vi "Colour Recognition.vi"() -> ()   [LabVIEW 2015]
uses:
  <vilib>/vision/NI_Vision_Development_Module.lvlib
  subVIs/Log Level Control.ctl
  subVIs/Led Control.ctl
  subVIs/Video Resolution Control.ctl
  subVIs/Video Format Control.ctl
  subVIs/Depth Format Control.ctl
  subVIs/Depth Resolution Control.ctl
panel:
  in  "Threshold 2":cluster{"Lower value":sgl, "Upper value":sgl}={"Lower value"=125.0, "Upper value"=160.0} {"Lower value" scale=0.0..255.0; "Upper value" scale=0.0..255.0}
  in  "Led Option":T1
  in  "tilt degree":i32
  in  "Video and Depth config":T6={"Video Resolution"=enum."FREENECT_RESOLUTION_MEDIUM", "Video Format"=enum."FREENECT_VIDEO_RGB", "Depth Format"=enum."FREENECT_DEPTH_11BIT", "Depth Resolution"=enum."FREENECT_RESOLUTION_MEDIUM"}
  in  "Reset Default Settings":bool
  in  "Threshold":cluster{"Lower value":sgl, "Upper value":sgl}={"Lower value"=125.0, "Upper value"=160.0} {"Lower value" scale=0.0..255.0; "Upper value" scale=0.0..255.0}
  in  "Color Recognition":enum16{"Blue", "Red"}(ring)
  out "Image Preview":T7(plugin-control)
  in  "Erosion Value":dbl=5.0
  out "Object Area":dbl
  in  "Area Limit":dbl=2000.0 format="%#_13g"
  out "Colour Matching":T7(plugin-control)
  in  "STOP":bool
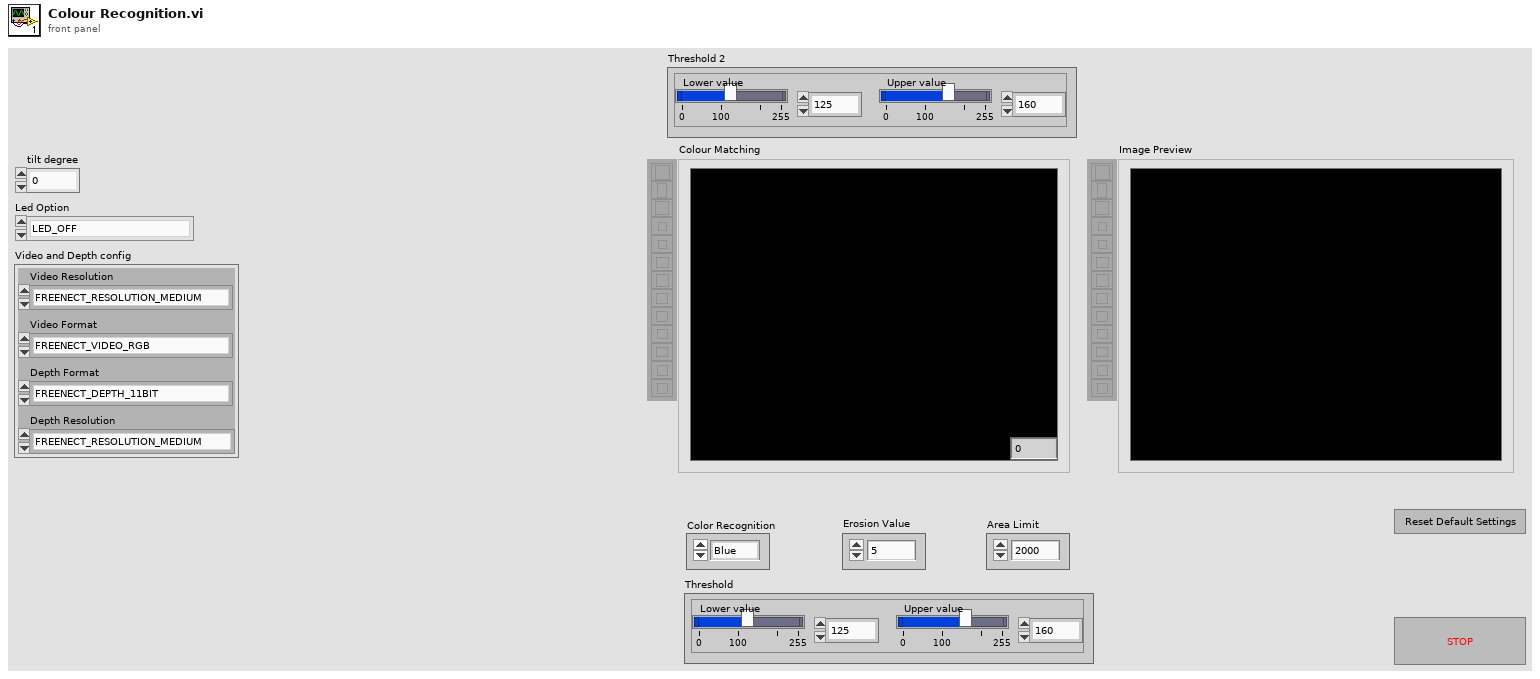
[diagram p1: front panel]
types:
  T1 = typedef "Led Control.ctl" = enum32{"LED_OFF", "LED_GREEN", "LED_RED", "LED_YELLOW", "LED_BLINK_GREEN", "LED_BLINK_GREEN2", "LED_BLINK_RED_YELLOW"}
  T2 = typedef "Video Resolution Control.ctl" = enum32{"FREENECT_RESOLUTION_LOW", "FREENECT_RESOLUTION_MEDIUM", "FREENECT_RESOLUTION_HIGH"}
  T3 = typedef "Video Format Control.ctl" = enum32{"FREENECT_VIDEO_RGB", "FREENECT_VIDEO_BAYER", "FREENECT_VIDEO_IR_8BIT", "FREENECT_VIDEO_IR_10BIT", "FREENECT_VIDEO_IR_10BIT_PACKED", "FREENECT_VIDEO_YUV_RGB", "FREENECT_VIDEO_YUV_RAW"}
  T4 = typedef "Depth Format Control.ctl" = enum32{"FREENECT_DEPTH_11BIT", "FREENECT_DEPTH_10BIT", "FREENECT_DEPTH_11BIT_PACKED", "FREENECT_DEPTH_10BIT_PACKED", "FREENECT_DEPTH_REGISTERED", "FREENECT_DEPTH_MM"}
  T5 = typedef "Depth Resolution Control.ctl" = enum16{"FREENECT_RESOLUTION_TINY", "FREENECT_RESOLUTION_LOW", "FREENECT_RESOLUTION_MEDIUM"}
  T6 = cluster{"Video Resolution":T2, "Video Format":T3, "Depth Format":T4, "Depth Resolution":T5}
  T7 = typedef "IMAQ Image.ctl" = refnum<image>
  T8 = typedef "Log Level Control.ctl" = enum32{"FREENECT_LOG_FATAL", "FREENECT_LOG_ERROR", "FREENECT_LOG_WARNING", "FREENECT_LOG_NOTICE", "FREENECT_LOG_INFO", "FREENECT_LOG_DEBUG", "FREENECT_LOG_SPEW", "FREENECT_LOG_FLOOD"}
  T9 = typedef "Particle Parameters" = i32
  T10 = cluster{"Numeric":dbl, "Numeric":dbl, "Numeric":dbl, "Numeric":dbl}
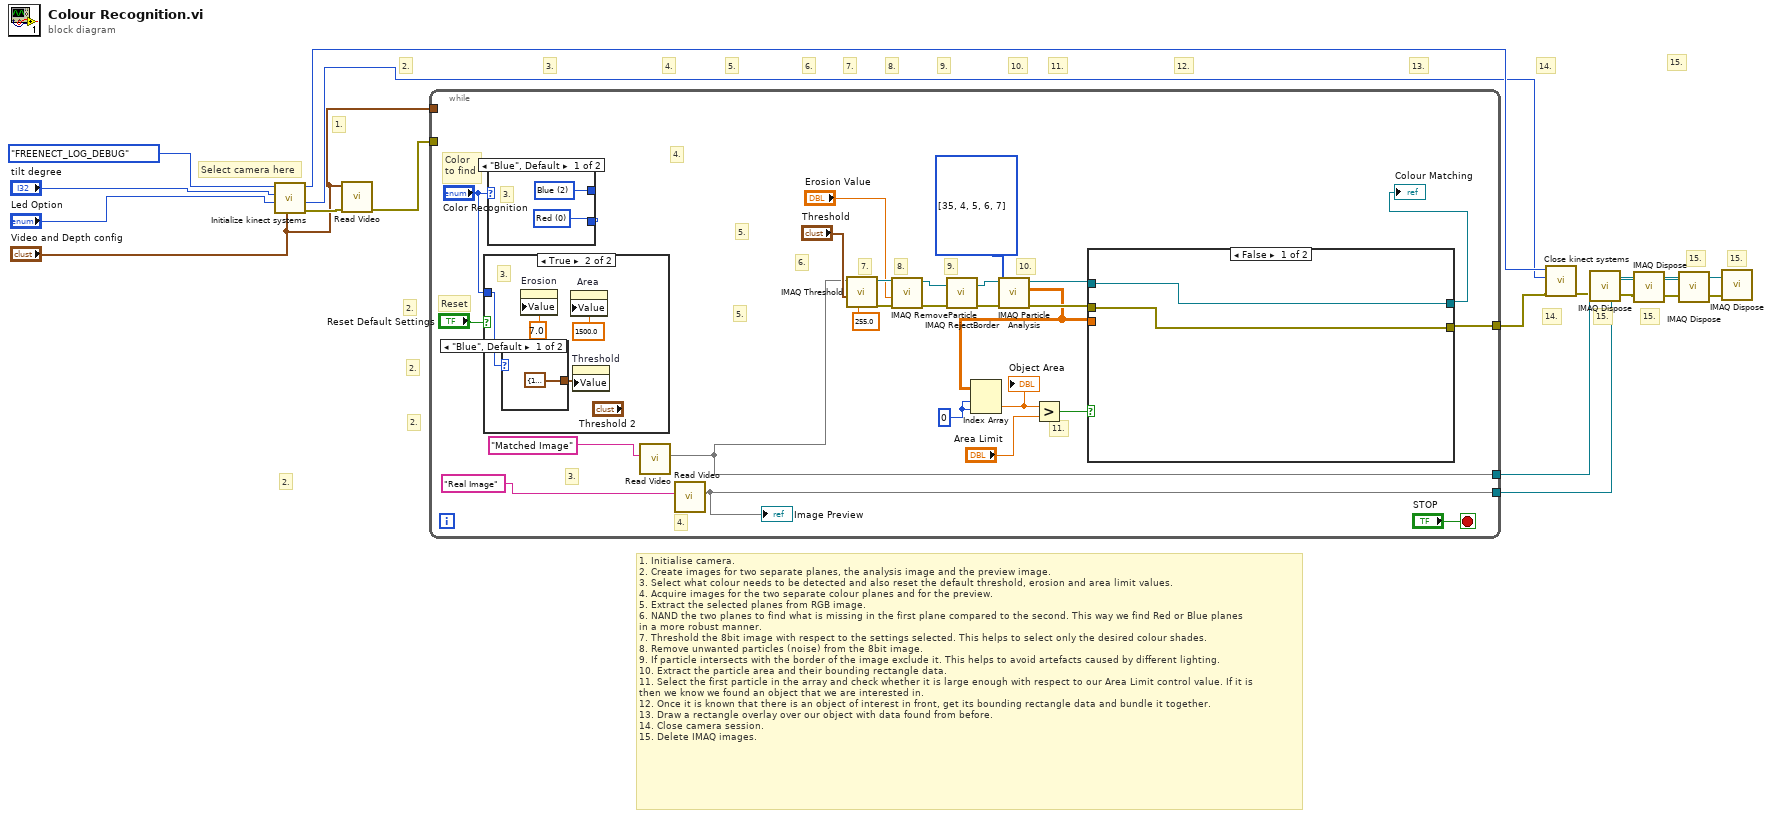
[diagram p0: block diagram]
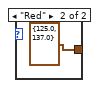
[diagram p3: hidden frame]
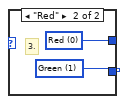
[diagram p4: hidden frame]
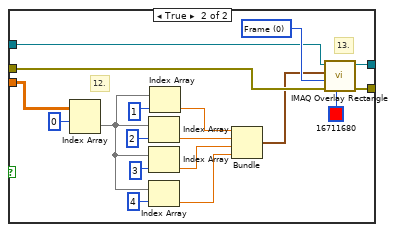
[diagram p5: hidden frame]
diagram:
  # "Select camera here"
  # "1. Initialise camera.\n2. Create images for two separate planes, the analysis image and the preview image.\n3. Select what colour needs to be detected and also reset the default threshold, erosion and area limit values.\n4. Acquire images for the two separate colour planes and for the preview.\n5. Extract the selected planes from RGB image.\n6. NAND the two planes to find what is missing in the first plane compared to the second. This way we find Red or Blue planes\nin a more robust manner.\n7. Threshold the 8bit image with respect to the settings selected. This helps to select only the desired colour shades.\n8. Remove unwanted particles (noise) from the 8bit image.\n9. If particle intersects with the border of the image exclude it. This helps to avoid artefacts caused by different lighting.\n10. Extract the particle area and their bounding rectangle data.\n11. Select the first particle in the array and check whether it is large enough with respect to our Area Limit control value. If it is\nthen we know we found an object that we are interested in.\n12. Once it is known that there is an object of interest in front, get its bounding rectangle data and bundle it together.\n13. Draw a rectangle overlay over our object with data found from before.\n14. Close camera session.\n15. Delete IMAQ images."
  # "15."
  # "15."
  # "15."
  # "15."
  # "15."
  # "14."
  # "14."
  # "13."
  # "12."
  # "11."
  # "10."
  # "2."
  # "2."
  # "2."
  # "2."
  # "9."
  # "8."
  # "7."
  # "6."
  # "5."
  # "4."
  # "3."
  # "2."
  # "1."
  n1 = call "Initialize kinect systems.vi"("Video and Depth config"="Video and Depth config", "Led Option"="Led Option", "tilt degree"="tilt degree", "Log Level"=Log_Level_Control."FREENECT_LOG_DEBUG") -> ("error out"=w3:errorcluster, "Kinect Handle"=w4:i64, "Video Handle out"=w5:i64)  [unwired: 4 in, 1 out]
  n2 = call "Read Video.vi"("error in (no error)"=w3, "input cluster"="Video and Depth config") -> ("error out"=w2:errorcluster)  [unwired: 7 in, 2 out]
  n3 = while {
    tunnel: w2 -> [_]
    tunnel: [w16] -> w13
    tunnel: [w26] -> w6
    tunnel: [w18] -> w11
    tunnel: "Video and Depth config" -> [_]
    stop <- "STOP" stop-if-true
    w37 = 0 ("index (row)")
    w39 = T9[] [35, 4, 5, 6, 7] items=["Center of Mass X", "Center of Mass Y", "First Pixel X", "First Pixel Y", "Bounding Rect Left", "Bounding Rect Top", "Bounding Rect Right", "Bounding Rect Bottom", "Max Feret Diameter Start X", "Max Feret Diameter Start Y", "Max Feret Diameter End X", "Max Feret Diameter End Y", "Max Horiz. Segment Length Left", "Max Horiz. Segment Length Right", "Max Horiz. Segment Length Row", "-", "Bounding Rect Width", "Bounding Rect Height", "Bounding Rect Diagonal", "Perimeter", "Convex Hull Perimeter", "Holes' Perimeter", "Max Feret Diameter", "Equivalent Ellipse Major Axis", "Equivalent Ellipse Minor Axis", "Equivalent Ellipse Minor Axis (Feret)", "Equivalent Rect Long Side", "Equivalent Rect Short Side", "Equivalent Rect Diagonal", "Equivalent Rect Short Side (Feret)", "Average Horiz. Segment Length", "Average Vert. Segment Length", "Hydraulic Radius", "Waddel Disk Diameter", "-", "Area", "Holes' Area", "Particle & Holes' Area", "Convex Hull Area", "Image Area", "-", "Number of Holes", "Number of Horiz. Segments", "Number of Vert. Segments", "-", "Orientation", "Max Feret Diameter Orientation", "-", "% Area/Image Area", "% Area/(Particle & Holes' Area)", "Ratio of Equivalent Ellipse Axes", "Ratio of Equivalent Rect Sides", "-", "Elongation Factor", "Compactness Factor", "Heywood Circularity Factor", "Type Factor", "-", "Sum X", "Sum Y", "Sum XX", "Sum XY", "Sum YY", "Sum XXX", "Sum XXY", "Sum XYY", "Sum YYY", "-", "Moment of Inertia XX", "Moment of Inertia XY", "Moment of Inertia YY", "Moment of Inertia XXX", "Moment of Inertia XXY", "Moment of Inertia XYY", "Moment of Inertia YYY", "Norm. Moment of Inertia XX", "Norm. Moment of Inertia XY", "Norm. Moment of Inertia YY", "Norm. Moment of Inertia XXX", "Norm. Moment of Inertia XXY", "Norm. Moment of Inertia XYY", "Norm. Moment of Inertia YYY", "Hu Moment 1", "Hu Moment 2", "Hu Moment 3", "Hu Moment 4", "Hu Moment 5", "Hu Moment 6", "Hu Moment 7"] ("Pixel Measurements")
    # "3."
    # "11."
    # "10."
    # "4."
    # "4."
    # "5."
    # "5."
    # "6."
    # "7."
    # "8."
    # "9."
    # "Reset"
    # "Color\nto find"
    n4 = case shown="True" "Reset Default Settings" {
      tunnel: "Color Recognition" -> [_ w45]
      frame False {
        # "3."
      }
      frame True {
        # "3."
        n5 = case shown="\"Blue\", Default" w45 {
          tunnel: [cluster{"Lower value":sgl, "Upper value":sgl} {"Lower value"=125.0, "Upper value"=160.0} ("Threshold Range") cluster{"Lower value":sgl, "Upper value":sgl} {"Lower value"=125.0, "Upper value"=137.0} ("Threshold Range")] -> w42
          frame "Blue", Default {
          }
          frame "Red" {
          }
        }
        n6 = property on="Erosion" class="DigNum (strict)"("Value"=7.0 ("Erosion Value")) -> ()  [unwired: 2 in, 2 out]
        n7 = property on="Area" class="DigNum (strict)"("Value"=1500.0 ("Area Limit")) -> ()  [unwired: 2 in, 2 out]
        n8 = property on="Threshold" class="Clust (strict)"("Value"=w42) -> ()  [unwired: 2 in, 2 out]
      }
    }
    n9 = case shown="\"Blue\", Default" "Color Recognition" {
      tunnel: [w49 w51] -> _
      tunnel: [w48 w50] -> _
      frame "Blue", Default {
        w48 = 0 items=["Red", "Green", "Blue", "Hue", "Saturation", "Luminance", "Value", "Intensity"] ("Color Plane")
        w49 = 2 items=["Red", "Green", "Blue", "Hue", "Saturation", "Luminance", "Value", "Intensity"] ("Color Plane")
        # "3."
      }
      frame "Red" {
        w50 = 1 items=["Red", "Green", "Blue", "Hue", "Saturation", "Luminance", "Value", "Intensity"] ("Color Plane")
        w51 = 0 items=["Red", "Green", "Blue", "Hue", "Saturation", "Luminance", "Value", "Intensity"] ("Color Plane")
        # "3."
      }
    }
    n10 = call "Read Video.vi"("Image Name"="Matched Image") -> (2:w16)  [unwired: 7 in, 3 out]
    n11 = call "Read Video.vi"("Image Name"="Real Image") -> (2:w18)  [unwired: 7 in, 3 out]
    "Image Preview" <- w18
    n12 = call "IMAQ Threshold"("Replace Value"=sgl 255.0, "Range"="Threshold", "Image Src"=w16) -> ("error out"=w32:errorcluster, "Image Dst Out"=w33:T7)  [unwired: 7 in]
    n13 = call "IMAQ RemoveParticle"("error in (no error)"=w32, "Number of Erosion"="Erosion Value", "Image Src"=w33) -> ("error out"=w31:errorcluster, "Image Dst Out"=w30:T7)  [unwired: 7 in]
    n14 = call "IMAQ RejectBorder"("error in (no error)"=w31, "Image Src"=w30) -> ("error out"=w28:errorcluster, "Image Dst Out"=w29:T7)  [unwired: 4 in]
    n15 = call "IMAQ Particle Analysis"("error in (no error)"=w28, "Pixel Measurements"=w39, "Image"=w29) -> ("error out"=w27:errorcluster, "Particle Measurements (Pixels)"=w25:dbl[][], "Image Out (duplicate)"=w38:T7)  [unwired: 3 in, 3 out]
    n16 = Index Array(array=w25, index (row)=w37, index (col)=w37) -> (element=w36:dbl)
    "Object Area" <- w36
    n17 = Greater?(x=w36, y="Area Limit") -> (0:w34:bool)
    n18 = case shown="False" w34 {
      tunnel: [w53 w70] -> w24
      tunnel: w38 -> [w53 w68]
      tunnel: w27 -> [w52 w64]
      tunnel: [w52 w67] -> w26
      tunnel: w25 -> [_ w66]
      frame False {
      }
      frame True {
        w69 = u32 0 items=["Frame", "Fill", "Highlight"] ("Drawing Mode (Frame)")
        # "13."
        # "12."
        n19 = Index Array(array=w66, index (row)=0) -> (element=w63:dbl[])  [unwired: 1 in]
        n20 = Index Array(array=w63, index=2) -> (element=w57:dbl)
        n21 = Index Array(array=w63, index=3) -> (element=w56:dbl)
        n22 = Index Array(array=w63, index=4) -> (element=w55:dbl)
        n23 = Index Array(array=w63, index=1) -> (element=w58:dbl)
        n24 = Bundle("Numeric"=w58, "Numeric"=w57, "Numeric"=w56, "Numeric"=w55) -> (w54:T10)  [unwired: 1 in]
        n25 = call "IMAQ Overlay Rectangle"("Color"=u32 16711680, "error in (no error)"=w64, "Drawing Mode (Frame)"=w69, "Rectangle"=w54, "Image"=w68) -> ("error out"=w67:errorcluster, "Image Out"=w70:T7)  [unwired: 5 in]
      }
    }
    "Colour Matching" <- w24
  }
  n26 = call "Close kinect systems.vi"("error in (no error)"=w6, "Kinect Handle"=w4, "Video handle in"=w5) -> ("error out"=w7:errorcluster)  [unwired: 8 in]
  n27 = call "IMAQ Dispose"("error in (no error)"=w7) -> ("error out"=w15:errorcluster)  [unwired: 2 in, 3 out]
  n28 = call "IMAQ Dispose"("error in (no error)"=w15) -> ("error out"=w14:errorcluster)  [unwired: 2 in, 3 out]
  n29 = call "IMAQ Dispose"("Image"=w13, "error in (no error)"=w14) -> ("error out"=w12:errorcluster)  [unwired: 1 in, 3 out]
  n30 = call "IMAQ Dispose"("Image"=w11, "error in (no error)"=w12) -> ()  [unwired: 1 in, 4 out]
